vi "Mean_and_Standard_Deviation.vi"(6 "Iterations":i32, 7 "Data Points":i32, 11 "2D array":dbl[][](array[numeric])) -> (0 "Standard Error":dbl[](array[numeric]), 1 "Standard Deviation":dbl[](array[numeric]), 3 "Mean":dbl[](array[numeric]))   [LabVIEW 2018]
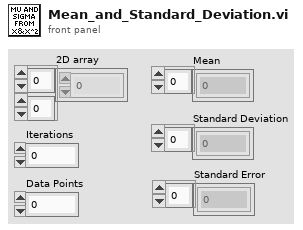
[diagram p1: front panel]
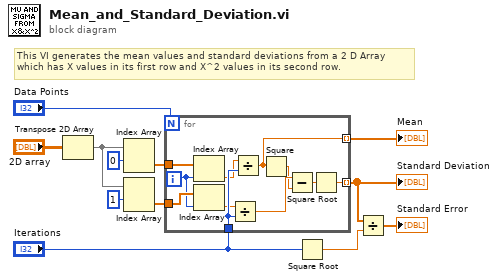
[diagram p0: block diagram]
diagram:
  # "This VI generates the mean values and standard deviations from a 2 D Array\nwhich has X values in its first row and X^2 values in its second row."
  n1 = Transpose 2D Array(2D array="2D array") -> (transposed array=w10:dbl[][])
  n2 = Index Array(array=w10, index (row)=0 ("index")) -> (element=w8:dbl[])  [unwired: 1 in]
  n3 = Index Array(array=w10, index (row)=1) -> (element=w7:dbl[])  [unwired: 1 in]
  n4 = for {
    N: "Data Points" -> [_]
    tunnel: w8 -> [w23]
    tunnel: w7 -> [w22]
    tunnel: "Iterations" -> [w17]
    tunnel: [w14] -> w9 mode=indexing
    tunnel: [w13] -> w3 mode=indexing
    i -> [w21]
    n5 = Index Array(array=w23, index=w21) -> (element=w16:dbl)
    n6 = Index Array(array=w22, index=w21) -> (element=w15:dbl)
    n7 = Divide(x=w15, y=w17) -> (x/y=w20:dbl)
    n8 = Divide(x=w16, y=w17) -> (x/y=w14:dbl)
    n9 = Square(x=w14) -> (x^2=w19:dbl)
    n10 = Subtract(x=w20, y=w19) -> (x-y=w18:dbl)
    n11 = Square Root(x=w18) -> (sqrt(x)=w13:dbl)
  }
  "Standard Deviation" <- w3
  "Mean" <- w9
  n12 = Square Root(x="Iterations") -> (sqrt(x)=w2:dbl)
  n13 = Divide(x=w3, y=w2) -> (x/y=→"Standard Error":dbl[])
